vi "reprocess orientation2.vi"(10 "orientation_model":u32(ring) items=["APDM_ORIENTATION_MODEL_ALL", "APDM_ORIENTATION_MODEL_NO_MAG", "APDM_ORIENTATION_MODEL_UNDISTURBED_MAG"], 11 "file_in":string) -> (2 "function return":i32, 3 "file_in out":string)   [LabVIEW 2019, in "apdm.lvlib"]
doc: "APDM_EXPORT int apdm_reprocess_orientation2(char *file_in, apdm_orientation_model_t orientation_model);"
uses:
  apdm.lvlib
  Lee Lab/CP FES Walking 2018/Code/Working/LabVIEW/apdm.dll
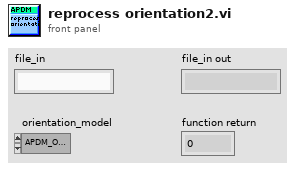
[diagram p1: front panel]
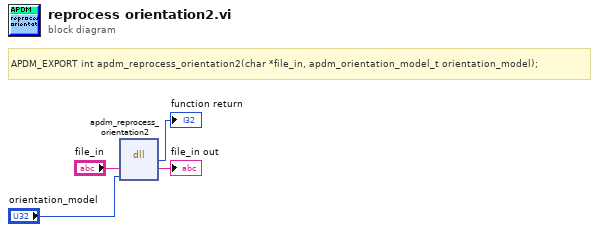
[diagram p0: block diagram]
diagram:
  # "APDM_EXPORT int apdm_reprocess_orientation2(char *file_in, apdm_orientation_model_t orientation_model);"
  n1 = dll-call lib="C:/Users/jfalesi/Dropbox/Lee Lab/CP FES Walking 2018/Code/Working/LabVIEW/apdm.*" fn="apdm_reprocess_orientation2"("file_in"="file_in", "orientation_model"="orientation_model") -> (→"function return":i32, "file_in"=→"file_in out":string)  [unwired: 4 in, 2 out]
